vi "map_frequency.vi"(11 "frequency":dbl) -> (3 "note":string)   [LabVIEW 2016]
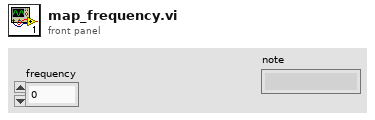
[diagram p1: front panel]
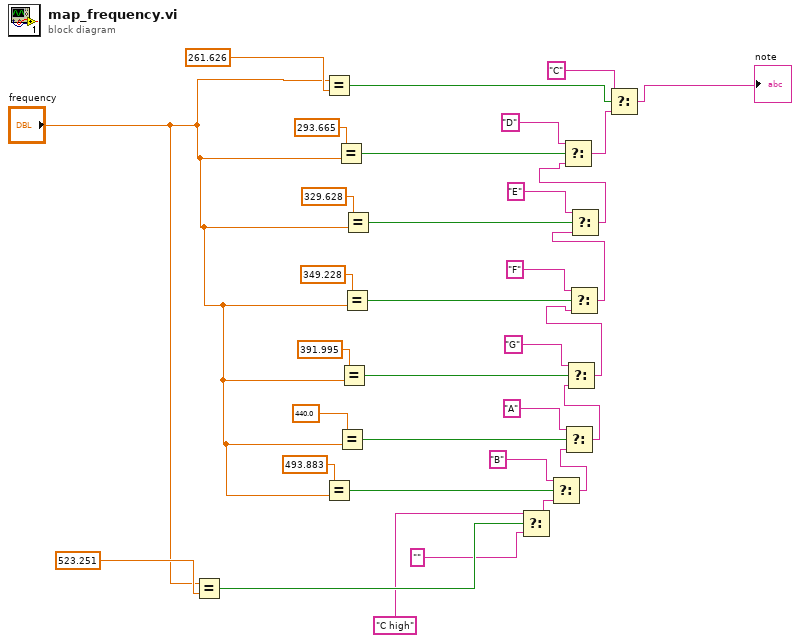
[diagram p0: block diagram]
diagram:
  n1 = Equal?(x="frequency", y=523.251) -> (x = y?=w6:bool)
  n2 = Equal?(x="frequency", y=261.626) -> (x = y?=w34:bool)
  n3 = Equal?(x=493.883, y="frequency") -> (x = y?=w9:bool)
  n4 = Equal?(x=293.665, y="frequency") -> (x = y?=w29:bool)
  n5 = Equal?(x=440.0, y="frequency") -> (x = y?=w13:bool)
  n6 = Equal?(x=391.995, y="frequency") -> (x = y?=w17:bool)
  n7 = Equal?(x=349.228, y="frequency") -> (x = y?=w21:bool)
  n8 = Equal?(x=329.628, y="frequency") -> (x = y?=w25:bool)
  n9 = Select(t="C high", s=w6, f="") -> (s? t:f=w1:string)
  n10 = Select(t="B", s=w9, f=w1) -> (s? t:f=w8:string)
  n11 = Select(t="A", s=w13, f=w8) -> (s? t:f=w12:string)
  n12 = Select(t="G", s=w17, f=w12) -> (s? t:f=w16:string)
  n13 = Select(t="F", s=w21, f=w16) -> (s? t:f=w20:string)
  n14 = Select(t="E", s=w25, f=w20) -> (s? t:f=w24:string)
  n15 = Select(t="D", s=w29, f=w24) -> (s? t:f=w28:string)
  n16 = Select(t="C", s=w34, f=w28) -> (s? t:f=→"note":string)
